vi "Error Handler.vi"(10 "error in":errorcluster, 11 "Queue in":refnum<queue>) -> (0 "error out":errorcluster, 3 "Queue out":refnum<queue>)   [LabVIEW 2019]
uses:
  MessageFormat1.ctl
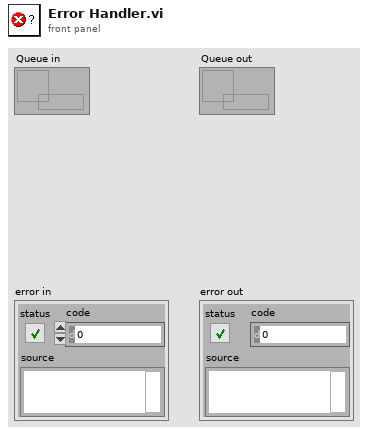
[diagram p1: front panel]
types:
  T1 = typedef "MessageFormat1.ctl" = cluster{"Consumer State":string, "RxData":string, "error constant":errorcluster, "Connected":bool, "Bool2":bool}
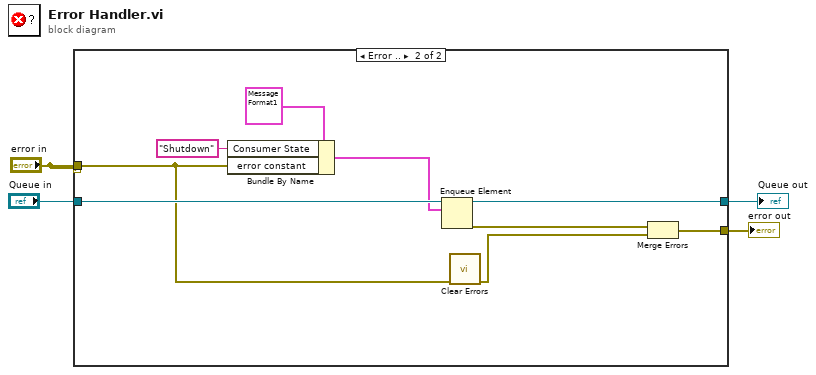
[diagram p0: block diagram]
diagram:
  n1 = case shown="Error .." "error in" {
    selector: "error in" -> [w5 _]
    tunnel: "error in" -> [_ w7]
    tunnel: "Queue in" -> [w6 w14]
    tunnel: [w6 w13] -> w2
    tunnel: [w5 w11] -> w3
    frame No Error {
    }
    frame Error {
      n2 = Bundle By Name(cluster=T1 {"Consumer State"="Consumer State", "RxData"="Received Data", "error constant"={"status"=FALSE, "code"=0, "source"=""}, "Connected"=FALSE, "Bool2"=FALSE} ("Queue Definition"), "Consumer State"="Shutdown", "error constant"=w7) -> (w12:T1)
      n3 = Enqueue Element(queue=w14, element=w12) -> (queue out=w13:refnum<queue>, error out=w10:errorcluster)  [unwired: 2 in, 1 out]
      n4 = call <vilib>:"Clear Errors.vi"("error in (no error)"=w7) -> ("error out"=w8:errorcluster)  [unwired: 5 in, 1 out]
      n5 = Merge Errors(w10, w8) -> (w11:errorcluster)
    }
  }
  "error out" <- w3
  "Queue out" <- w2
